vi "Przenies mnozniki FVG.vi"(7 "Akcja (Get)":T2, 8 "error in (no error)":errorcluster, 9 "AI A_B params in":T1, 10 "DI Mnozniki in":dbl[](array[numeric]), 11 "AI Mnozniki in":dbl[](array[numeric])) -> (0 "error out":errorcluster, 1 "AI A_B params out":T1, 2 "DI Mnozniki out":dbl[](array[numeric]), 3 "AI Mnozniki out":dbl[](array[numeric]))   [LabVIEW 2014]
doc: "Zapamiętuje i przenosi mnożniki z pętli GUI do akwizycji"
uses:
  Kontrolki/FVGs/FVG GUI akcje.ctl
  Kontrolki/GUI/HW_A_B_params .ctl
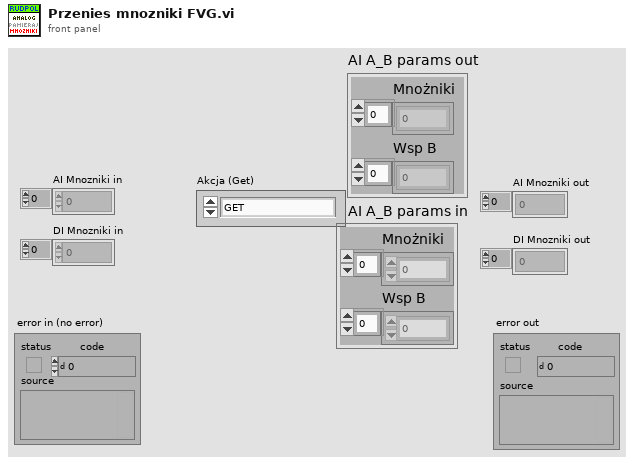
[diagram p1: front panel]
types:
  T1 = typedef "HW_A_B_params .ctl" = cluster{"Mnożniki":dbl[], "Wsp B":dbl[]}
  T2 = typedef "FVG GUI akcje.ctl" = enum16{"GET", "SET AI Aktywny", "SET DI Aktywny"}
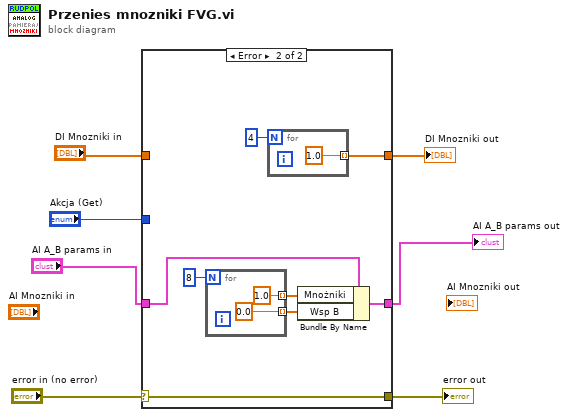
[diagram p0: block diagram]
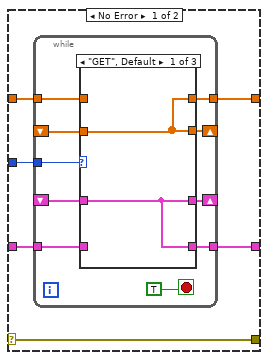
[diagram p2: hidden frame]
diagram:
  n1 = case shown="Error" "error in (no error)" {
    selector: "error in (no error)" -> [w13 w37]
    tunnel: [w13 w37] -> w6
    tunnel: "AI A_B params in" -> [w12 w33]
    tunnel: [w11 w32] -> w2
    tunnel: "DI Mnozniki in" -> [w10 _]
    tunnel: "Akcja (Get)" -> [w9 _]
    tunnel: [w8 w34] -> w3
    frame No Error {
      n2 = while {
        tunnel: w9 -> [w22]
        tunnel: w12 -> [w21]
        shift-right: [w20] -> _
        shift-left: _ -> [w19]
        tunnel: [w18] -> w11
        tunnel: w10 -> [w17]
        shift-right: [w16] -> _
        shift-left: _ -> [w14]
        tunnel: [w15] -> w8
        stop <- TRUE stop-if-true
        n3 = case shown="\"GET\", Default" w22 {
          tunnel: w21 -> [_ w27 _]
          tunnel: [w25 w27 w29] -> w20
          tunnel: w19 -> [w25 _ w29]
          tunnel: [w25 w27 w29] -> w18
          tunnel: w17 -> [_ _ w28]
          tunnel: [w24 w26 w28] -> w16
          tunnel: [w24 w26 w28] -> w15
          tunnel: w14 -> [w24 w26 _]
          frame "GET", Default {
          }
          frame "SET AI Aktywny" {
          }
          frame "SET DI Aktywny" {
          }
        }
      }
    }
    frame Error {
      n4 = for {
        N: 8 -> [_]
        tunnel: [1.0] -> w31 mode=indexing
        tunnel: [0.0] -> w30 mode=indexing
      }
      n5 = for {
        N: 4 -> [_]
        tunnel: [1.0] -> w34 mode=indexing
      }
      n6 = Bundle By Name(cluster=w33, "Mnożniki"=w31, "Wsp B"=w30) -> (w32:T1)
    }
  }
  "error out" <- w6
  "DI Mnozniki out" <- w3
  "AI A_B params out" <- w2
